vi "SP Convert Start Stop - Center Span.vi"(8 "Stop/Span In":dbl=1500.0, 9 "Start/Center In":dbl=500.0, 10 "Freq Format From":T1, 11 "Freq Format To":T1=enum."Center/Span") -> (0 "Stop/Span Out":dbl, 1 "Start/Center Out":dbl, 2 "Freq Format":T1)   [LabVIEW 2011]
uses:
  TypeDefs/SP Frequency Format.ctl
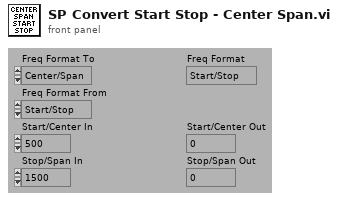
[diagram p1: front panel]
types:
  T1 = typedef "SP Frequency Format.ctl" = enum16{"Start/Stop", "Center/Span"}
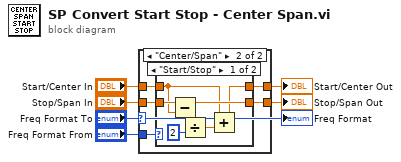
[diagram p0: block diagram]
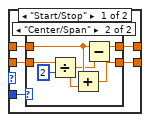
[diagram p2: hidden frame]
diagram:
  n1 = case shown="\"Center/Span\"" "Freq Format To" {
    tunnel: "Stop/Span In" -> [w11 w24]
    tunnel: "Start/Center In" -> [w10 w23]
    tunnel: "Freq Format From" -> [w9 w22]
    tunnel: [w8 w21] -> w2
    tunnel: [w7 w20] -> w3
    frame "Start/Stop" {
      n2 = case shown="\"Center/Span\"" w9 {
        tunnel: w11 -> [w12 w19]
        tunnel: w10 -> [w13 w17]
        tunnel: [w13 w14] -> w7
        tunnel: [w12 w15] -> w8
        frame "Start/Stop" {
        }
        frame "Center/Span" {
          n3 = Divide(x=w19, y=i8 2) -> (x/y=w16:dbl)
          n4 = Add(x=w17, y=w16) -> (x+y=w15:dbl)
          n5 = Subtract(x=w17, y=w16) -> (x-y=w14:dbl)
        }
      }
    }
    frame "Center/Span" {
      n6 = case shown="\"Start/Stop\"" w22 {
        tunnel: w24 -> [w30 w31]
        tunnel: w23 -> [w26 w32]
        tunnel: [w25 w32] -> w20
        tunnel: [w28 w31] -> w21
        frame "Start/Stop" {
          n7 = Subtract(x=w30, y=w26) -> (x-y=w28:dbl)
          n8 = Divide(x=w28, y=i8 2) -> (x/y=w27:dbl)
          n9 = Add(x=w26, y=w27) -> (x+y=w25:dbl)
        }
        frame "Center/Span" {
        }
      }
    }
  }
  "Stop/Span Out" <- w2
  "Start/Center Out" <- w3
  "Freq Format" <- "Freq Format To"
